vi "ChromaAcLoad.vi"() -> ()   [LabVIEW 2018, in "Visualization.lvlib" / "VisualizeAcPwr.lvclass"]
doc: "This VI listens for any measurement data associated with the provided PluginName and displays it to the user for analysis. The display is only suitable for data coming from the RoomAlert Plugin."
uses:
  VisualizeAcPwr.lvclass
  ChromaPowerSupply/Loop Parameters.ctl
  VisualizeBase/VisualizeBase_class/SubVIs/VisualizationOptions.ctl
  <vilib>/Utility/miscctls.llb/LVRectTypeDef.ctl
  AcPwr/AcPwrPlugins/ChromaAcLoadClass/TypeDefs/Device(s)Settings.ctl
  AcPwr/AcPwrPlugins/ChromaAcLoadClass/TypeDefs/ConfigMode.ctl
  AcPwr/AcPwrPlugins/ChromaAcLoadClass/TypeDefs/Measurements.ctl
  AcPwr/AcPwrPlugins/ChromaAcLoadClass/TypeDefs/MeasurementType.ctl
  AcPwr/AcPwrShared/clMeasurmentData.ctl
  AcPwr/AcPwrPlugins/AcPwrBaseClass/TypeDefs/SetParameterInputs.ctl
  <vilib>/event_ctls.llb/usereventprio.ctl
  VisualizeBase/VisualizeBase_class/Requests/VisUserEventType.ctl
  <extravilib>/ChannelInstances/Tag-bool/Write With Abort.vi
  <extravilib>/ChannelInstances/Tag-bool/Read With Abort.vi
  <extravilib>/ChannelInstances/Tag-bool/Instantiate.vi
  <extravilib>/ChannelInstances/Tag-bool/EndpointRead.vi
  <vilib>/Utility/error.llb/Error Cluster From Error Code.vi
  <extravilib>/ChannelInstances/Tag-bool/Endpoint.vi
  <vilib>/ErrorRing/Error Ring.xnode
  <userlib>/NIST/NISTErrorLib/NISTErrorLib.lvlib
  VisualizeBase/VisualizeBase_class/VisualizeBase.lvclass
  <extravilib>/ChannelInstances/Tag-bool.lvlib
  TestClass/Test.lvclass
  Sensor/VisualizeSensor.lvclass
  StatusAndLog/VisualizeStatus.lvclass
  AcPwr/AcPwrShared/AcPwrShared.lvlib
  AcPwr/AcPwrModule/AcPwrModule.lvlib
  AcPwr/AcPwrPlugins/ChromaAcLoadClass/ChromaAcLoad.lvclass
  AcPwr/AcPwrPlugins/AcPwrPlugins.lvlib
  AcPwr/AcPwrPlugins/AcPwrBaseClass/AcPwrBase.lvclass
panel:
  out "Chart#":i32
  out "MeasChannels":string[](array[string])
  out "Writetime":u32 caption="Sample Write Time(ms)"
  out "ExitHelperLoops?":bool
  out "CurrentType":string
  in  "Display":enum16{"Raw Data", "Voltage Vs Current"}(ring)
  in  "btnPause":bool
  in  "INIFilePath":path
  in  "ModuleID":i32
  in  "Log Data":bool=TRUE
  in  "btnStop":bool
  in  "btnReset":bool
  in  "btnClearTest":bool
  in  "btnStopModule":bool
  out "XY Graph":cluster{dbl[], dbl[]}(graph)
  out "Chart":waveform(dbl)[](graph)=[{"t0"=timestamp(3657200531.6397257 s since 1904-01-01), "dt"=1.0, "Y"=[46.19]}, {"t0"=timestamp(3657200531.6397257 s since 1904-01-01), "dt"=1.0, "Y"=[2.0]}, {"t0"=timestamp(3657200531.6397257 s since 1904-01-01), "dt"=1.0, "Y"=[60.0]}]
  in  "Device ON?":bool=TRUE
  in  "Resistance":bool
  in  "Power":bool
  in  "Current":bool
  in  "Voltage":bool
  in  "Resistance (Ohms)":dbl
  in  "Power (W)":dbl
  in  "Current (A)":dbl
  in  "Voltage (V)":dbl
  in  "btnRunParamLoop":bool
  in  "btnStopParameterLoop":bool
  in  "Loop Parameters":T1={"Parameter"=enum."Voltage", "Start Value"=5.0, "Increment"=1.0, "Interval (s)"=3.0, "# Iterations"=6, "End Value"=10.0} {"# Iterations" min=1; "Increment" format="%#.4f"}
  out "ErrorArray":errorcluster[](array[cluster])
  out "Incorrect DataType?":bool
  out "String Results":string
  in  "PluginName":string="Sensor.RoomAlert1"
  # "Set Parameter"
  # "Parameter Looping"
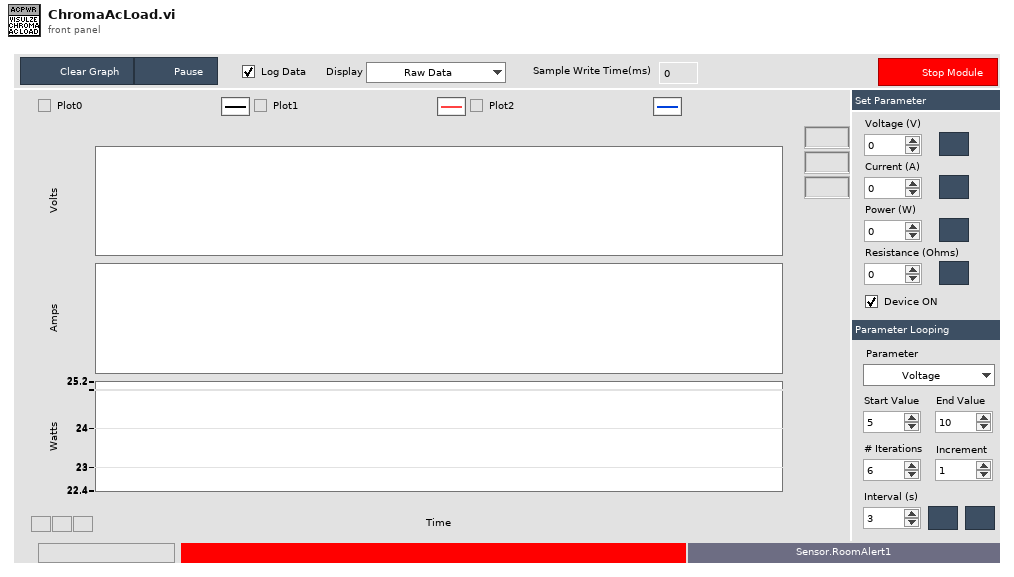
[diagram p1: front panel]
types:
  T1 = typedef "Loop Parameters.ctl" = cluster{"Parameter":enum16{"Voltage", "Current", "Power", "Resistance"}, "Start Value":dbl, "Increment":dbl, "Interval (s)":dbl, "# Iterations":u32, "End Value":dbl}
  T2 = typedef "Visualization.lvlib/VisualizeBase.lvclass/VisualizationOptions.ctl" = cluster{"PauseAtStartup":bool, "LogData":bool, "LaunchInSubPanel":bool, "FPMonitor":u16, "FPWindowBounds":T3, "MonitorBounds":cluster{"Left":i16, "Top":i16, "Right":i16, "Bottom":i16}, "MeasIndices":i32[]}
  T3 = typedef "LVRectTypeDef.ctl" = cluster{"Left":i16, "Top":i16, "Right":i16, "Bottom":i16}
  T4 = enum16{"open", "open or create", "create or replace", "create", "open (read-only)"}
  T5 = typedef "Visualization.lvlib/VisualizeBase.lvclass/VisRequestEvents.ctl" = cluster{"StopRequest":refnum<user-event>, "ResetRequest":refnum<user-event>, "FP Pop In or Out":refnum<user-event>}
  T6 = typedef "AcPwrShared.lvlib/AcPwrBroadcastEvents.ctl" = cluster{"DidInit":refnum<user-event>, "StatusUpdate":refnum<user-event>, "ErrorReport":refnum<user-event>, "DidStop":refnum<user-event>, "PathToINI":refnum<user-event>, "Measurements":refnum<user-event>, "LoadConfigFile":refnum<user-event>, "GetSettings":refnum<user-event>, "SetSettings":refnum<user-event>, "GetType&ID":refnum<user-event>, "GotSettings":refnum<user-event>, "GotSettingsLV":refnum<user-event>, "ParameterSet":refnum<user-event>}
  T7 = typedef "Visualization.lvlib/VisualizeBase.lvclass/VisFrmWrkBroadcastEvents.ctl" = cluster{"StatusUpdate":refnum<user-event>, "DidStop":refnum<user-event>, "NewModuleLoaded":refnum<user-event>, "StopVisualization":refnum<user-event>}
  T8 = typedef "AcPwrPlugins.lvlib/ChromaAcLoad.lvclass/Device(s)Settings.ctl" = cluster{"Configuration Mode":T9, "Phases":cluster{"Handle":string, "Name":string, "Phase Select":i32, "Instrument Options":string, "id query (T)":bool, "reset device (T)":bool, "Load Short Circuited":bool, "Line Synchronization":bool, "Load Current (A/Arms)":dbl, "Load Voltage (V/Vrms)":dbl, "Load Power (W)":dbl, "Load Resistance (Ohms)":dbl, "Load Current Peak Limit (A)":dbl, "Load Current Limit (A/Arms)":dbl, "Load Power Limit (W)":dbl, "Synch Frequency (Hz)":dbl, "Priority":enum16{"CF Only", "PF Only", "Both (CF)", "Both (PF)"}, "Crest Factor":dbl, "Power Factor":dbl, "Slew Rate":cluster{"Rise Slew Rate (A/ms)":i32, "Fall Slew Rate (A/ms)":i32}, "LC/RLC Mode":cluster{"Capacitance (uF)":i32, "Inductance (uH)":i32, "Series Resistance (Ohm)":dbl, "Parallel Resistance (Ohm)":dbl}, "Timing":cluster{"TimingOn":enum16{""}, "Hours":u32, "Minutes":u32, "Seconds":dbl, "CutoffVoltage":dbl}, "Connected":bool}[], "MeasName":string}
  T9 = typedef "AcPwrPlugins.lvlib/ChromaAcLoad.lvclass/ConfigMode.ctl" = enum16{"Constant Voltage (DC)", "Constant Power (DC)", "Constant Power (AC)", "Constant Current (DC)", "Constant Current (AC)", "Constant Resistance (DC)", "Constant Resistance (AC)", "Rectified Mode (DC)", "Inrush (AC)", "RLC CP (AC)", "RLC (AC)"}
  T10 = typedef "AcPwrPlugins.lvlib/ChromaAcLoad.lvclass/Measurements.ctl" = cluster{"Handle":string, "Name":string, "Enabled":bool, "Measurement Value":dbl, "Hold Peak Current Measurement":bool, "btnMeasFetch":bool, "ProtectionStatusString":string, "Measurement Type":T11}[]
  T11 = typedef "AcPwrPlugins.lvlib/ChromaAcLoad.lvclass/MeasurementType.ctl" = enum16{"Voltage (Vrms or V)", "Current (Arms or A)", "Power (W)", "Peak Voltage (V)", "Peak Current (A)", "Peak Power (W)", "Frequency (Hz)", "Resistance (Ohms)", "Voltage Overshoot (V)", "Positive Peak Current (A)", "Voltage Undershoot (V)", "Negative Peak Current (A)", "Apparent Power (VA)", "Reacitive Power (VAR)", "Voltage THD", "Power Factor", "Current's Crest Factor"}
  T12 = typedef "AcPwrShared.lvlib/clMeasurmentData.ctl" = cluster{"MeasName":string, "XML Data":string, "WaveformData":waveform(dbl)[]}
  T13 = typedef "AcPwrPlugins.lvlib/AcPwrBase.lvclass/SetParameterInputs.ctl" = cluster{"Type":string, "Parameter":string, "Phase":i32, "Value":dbl, "Command":string, "Time Stamp":timestamp}
  T14 = typedef "Visualization.lvlib/VisualizeBase.lvclass/VisUserEventType.ctl" = cluster{"BusIndex":i8, "Data":variant}
  T15 = typedef "usereventprio.ctl" = enum32{"high priority", "normal priority"}
  T16 = cluster{"Handle":string, "Name":string, "Phase Select":i32, "Instrument Options":string, "id query (T)":bool, "reset device (T)":bool, "Load Short Circuited":bool, "Line Synchronization":bool, "Load Current (A/Arms)":dbl, "Load Voltage (V/Vrms)":dbl, "Load Power (W)":dbl, "Load Resistance (Ohms)":dbl, "Load Current Peak Limit (A)":dbl, "Load Current Limit (A/Arms)":dbl, "Load Power Limit (W)":dbl, "Synch Frequency (Hz)":dbl, "Priority":enum16{"CF Only", "PF Only", "Both (CF)", "Both (PF)"}, "Crest Factor":dbl, "Power Factor":dbl, "Slew Rate":cluster{"Rise Slew Rate (A/ms)":i32, "Fall Slew Rate (A/ms)":i32}, "LC/RLC Mode":cluster{"Capacitance (uF)":i32, "Inductance (uH)":i32, "Series Resistance (Ohm)":dbl, "Parallel Resistance (Ohm)":dbl}, "Timing":cluster{"TimingOn":enum16{""}, "Hours":u32, "Minutes":u32, "Seconds":dbl, "CutoffVoltage":dbl}, "Connected":bool}[]
  T17 = cluster{"Handle":string, "Name":string, "Phase Select":i32, "Instrument Options":string, "id query (T)":bool, "reset device (T)":bool, "Load Short Circuited":bool, "Line Synchronization":bool, "Load Current (A/Arms)":dbl, "Load Voltage (V/Vrms)":dbl, "Load Power (W)":dbl, "Load Resistance (Ohms)":dbl, "Load Current Peak Limit (A)":dbl, "Load Current Limit (A/Arms)":dbl, "Load Power Limit (W)":dbl, "Synch Frequency (Hz)":dbl, "Priority":enum16{"CF Only", "PF Only", "Both (CF)", "Both (PF)"}, "Crest Factor":dbl, "Power Factor":dbl, "Slew Rate":cluster{"Rise Slew Rate (A/ms)":i32, "Fall Slew Rate (A/ms)":i32}, "LC/RLC Mode":cluster{"Capacitance (uF)":i32, "Inductance (uH)":i32, "Series Resistance (Ohm)":dbl, "Parallel Resistance (Ohm)":dbl}, "Timing":cluster{"TimingOn":enum16{""}, "Hours":u32, "Minutes":u32, "Seconds":dbl, "CutoffVoltage":dbl}, "Connected":bool}
  T18 = typedef "Tag-bool.lvlib/))Channel.ctl" = refnum<queue>
  T19 = typedef "sizeaction.ctl" = enum32{"Minimized", "Maximized", "Resized"}
  T20 = typedef "LVPoint32TypeDef.ctl" = cluster{"Horizontal":i32, "Vertical":i32}
  T21 = enum16{"Voltage", "Current", "Power", "Resistance"}
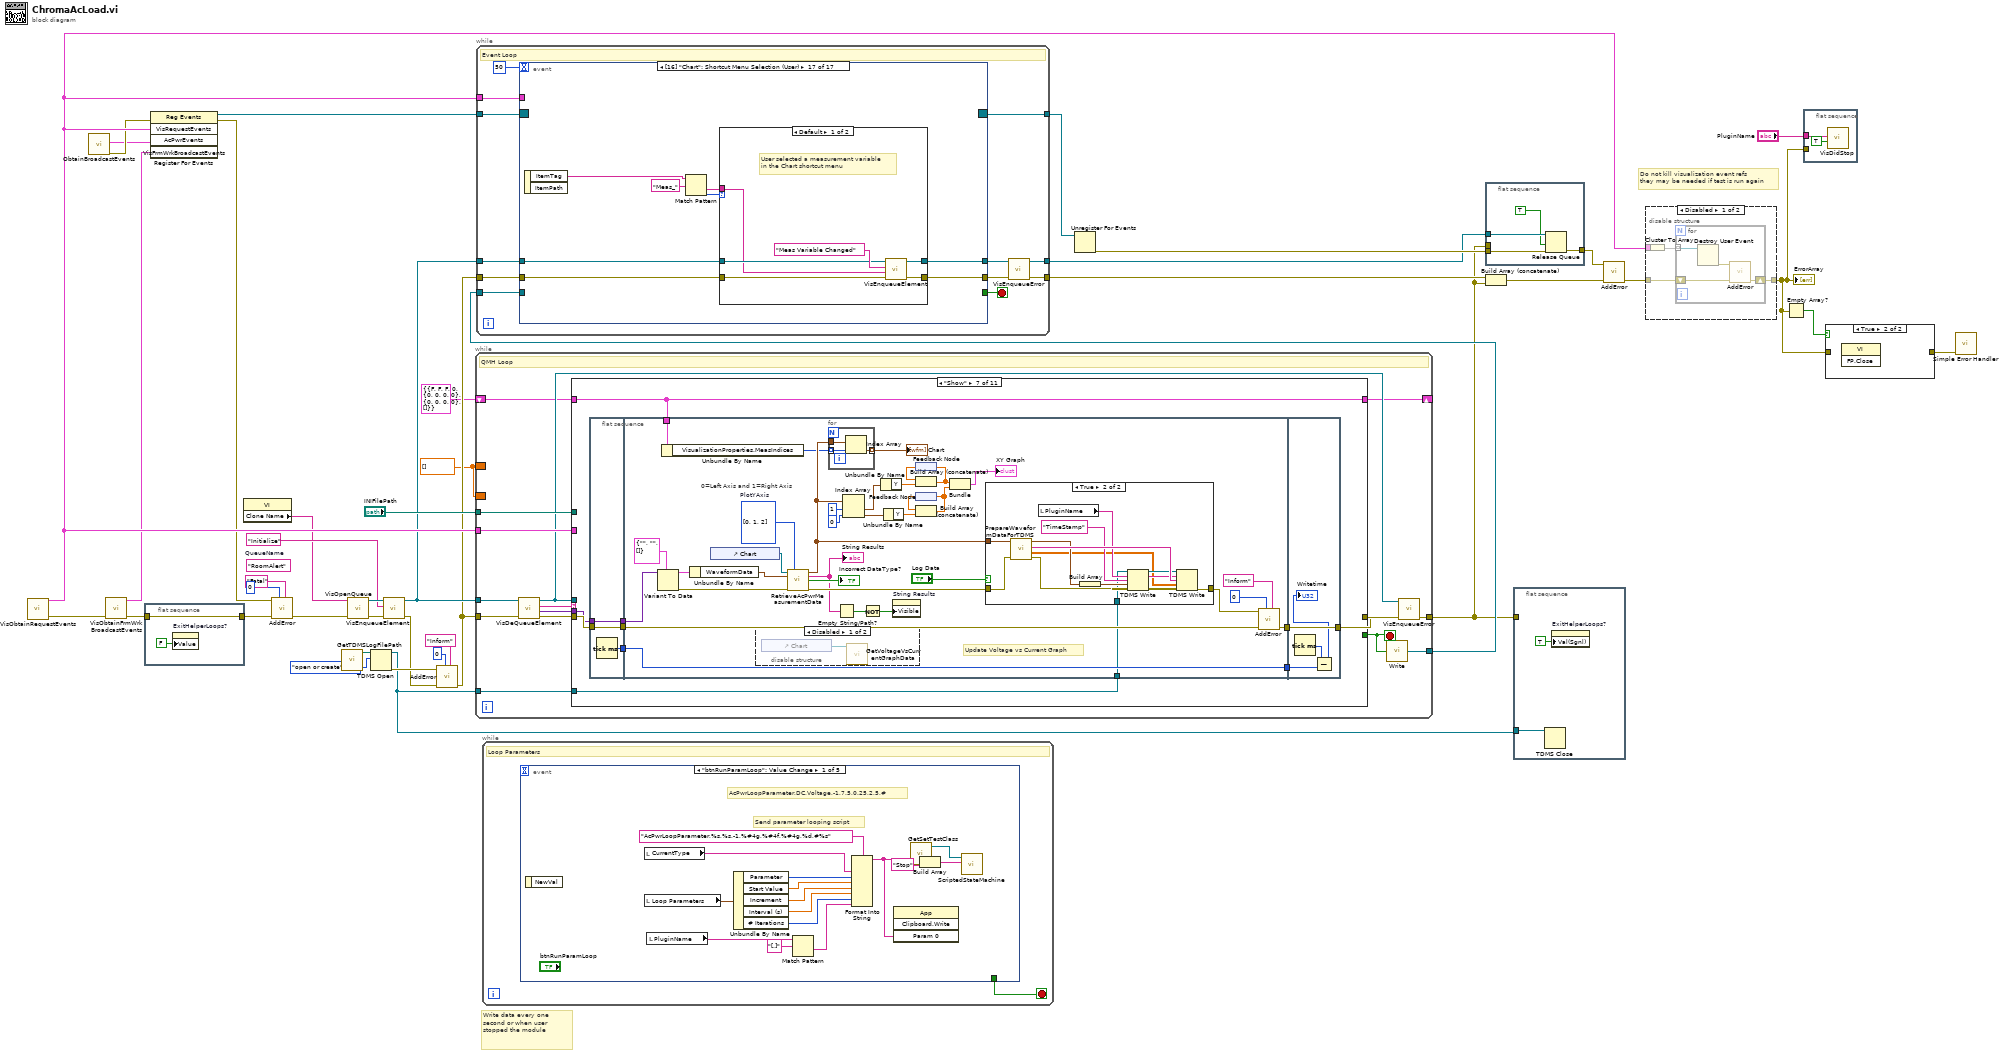
[diagram p0: block diagram]
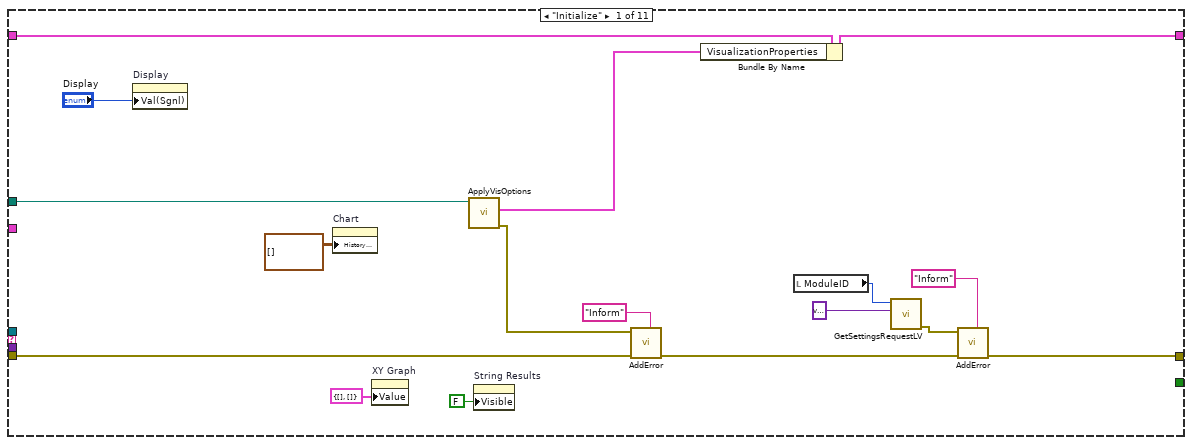
[diagram p2: hidden frame]
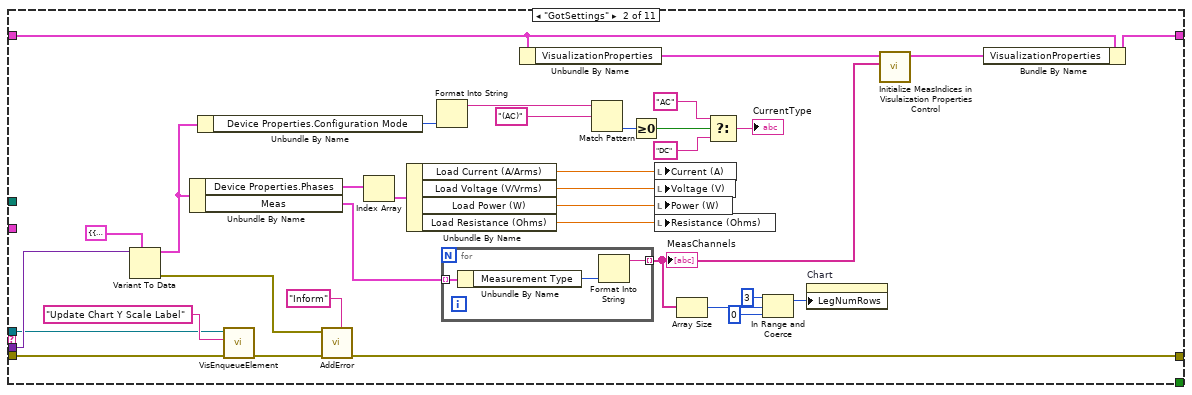
[diagram p3: hidden frame]
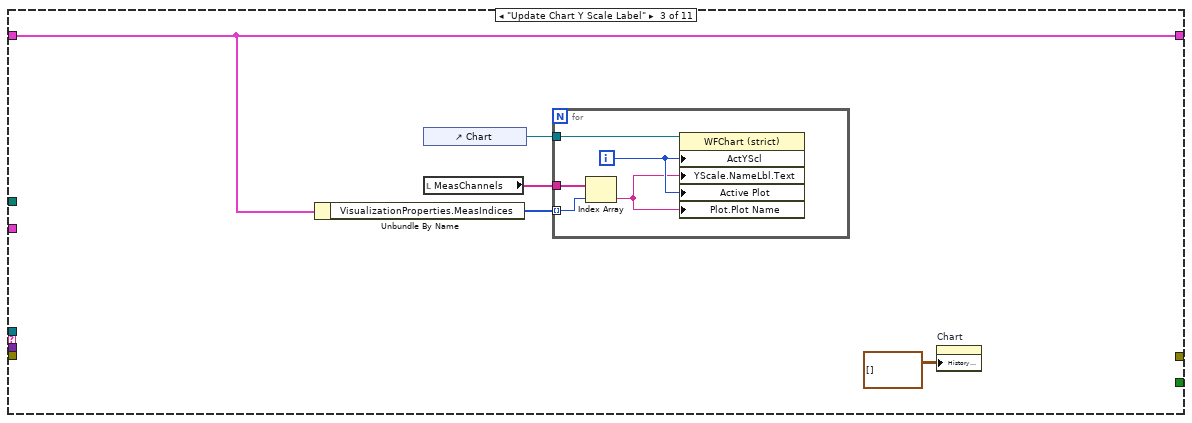
[diagram p4: hidden frame]
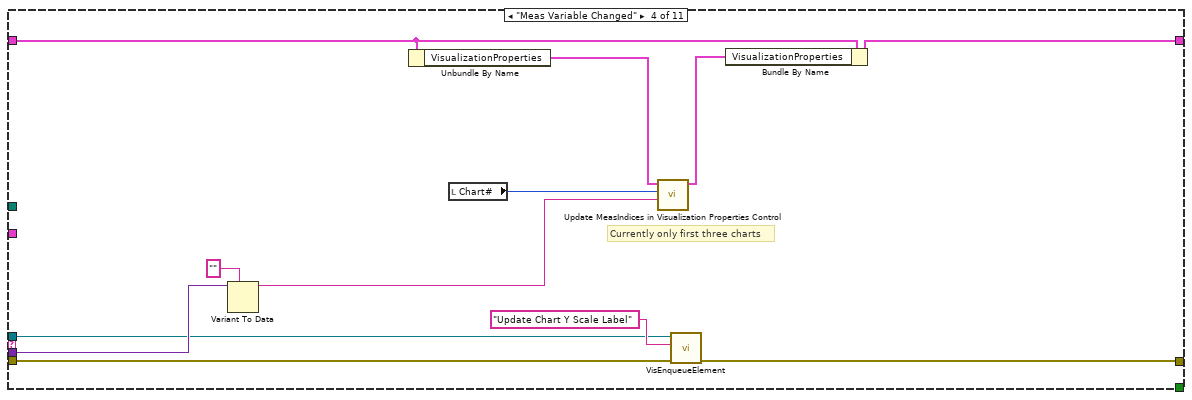
[diagram p5: hidden frame]
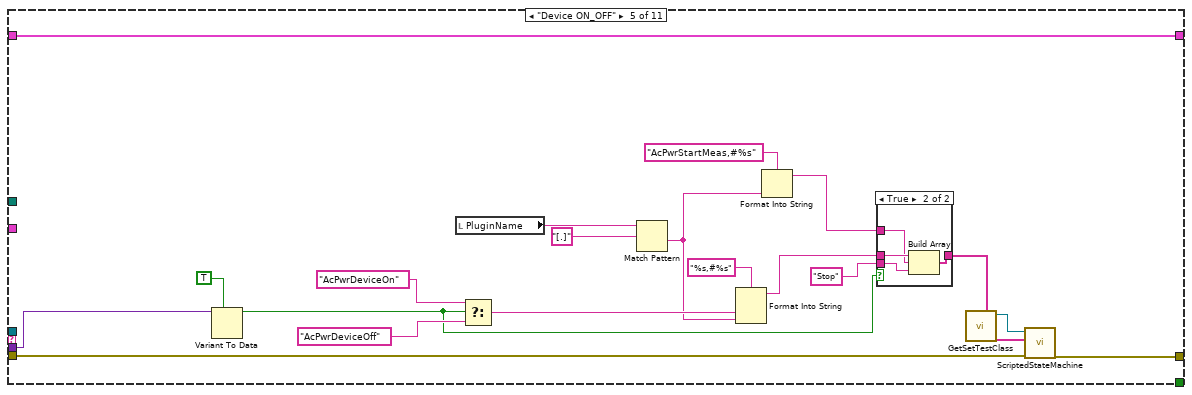
[diagram p6: hidden frame]
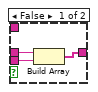
[diagram p7: hidden frame]
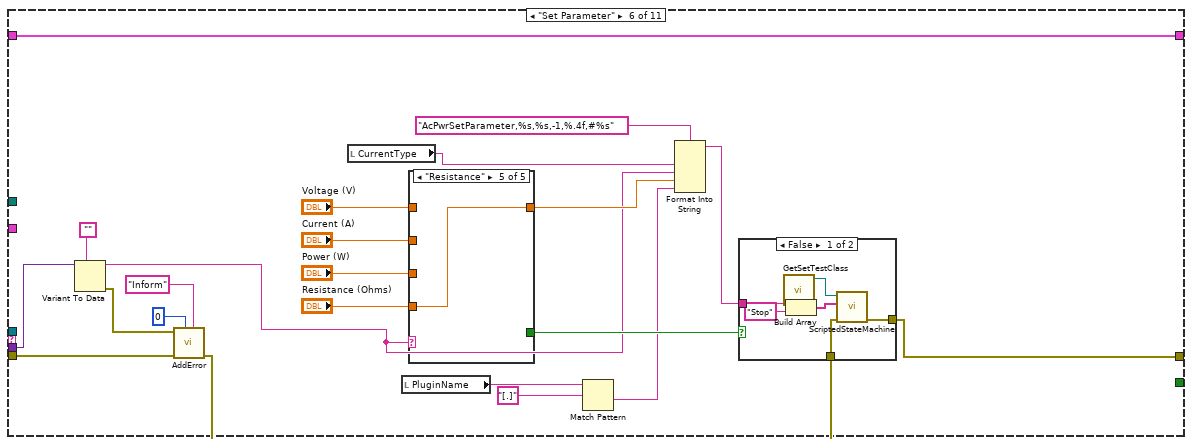
[diagram p8: hidden frame]
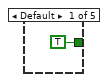
[diagram p10: hidden frame]
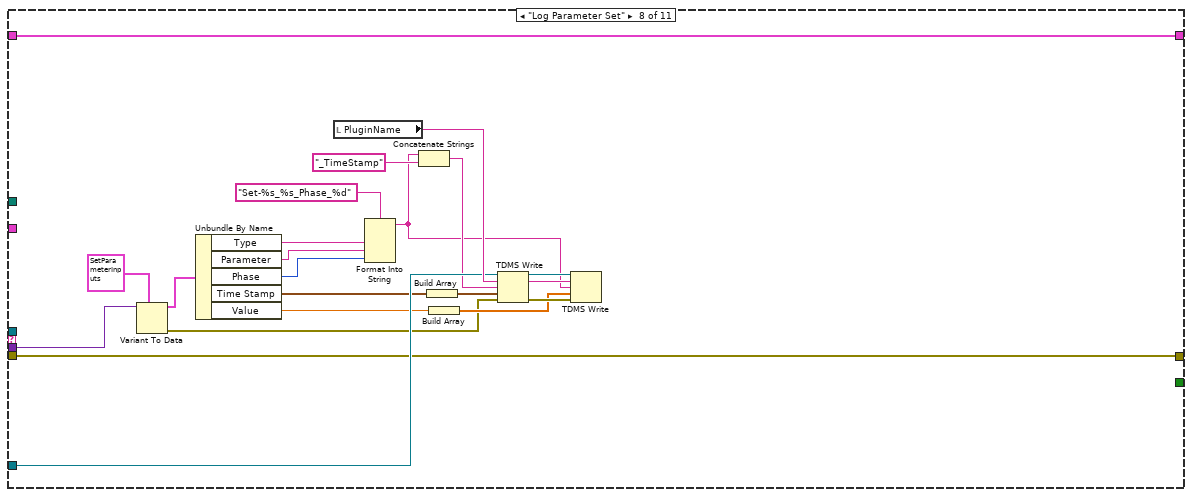
[diagram p16: hidden frame]
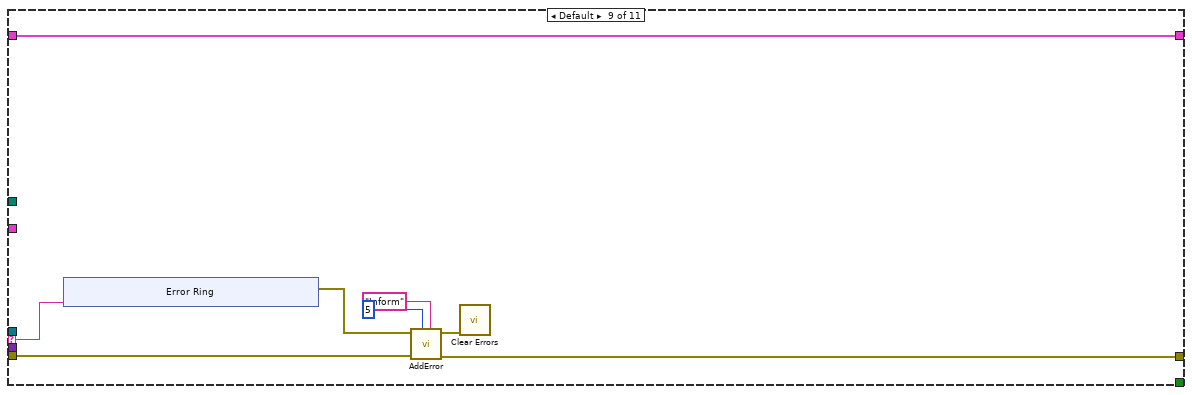
[diagram p17: hidden frame]
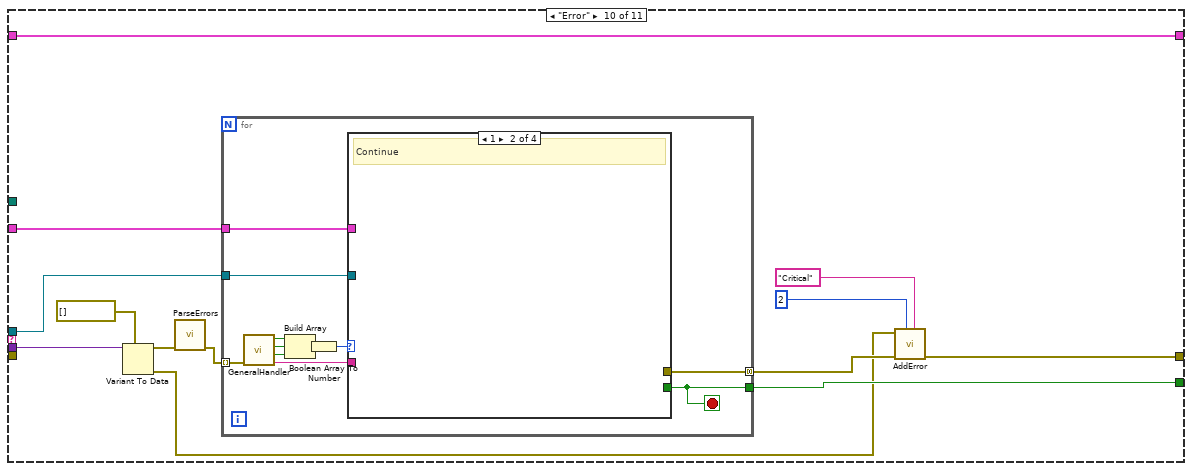
[diagram p18: hidden frame]
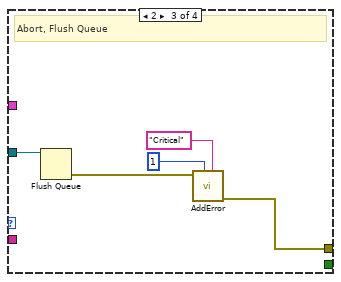
[diagram p20: hidden frame]
diagram:
  w3 = dbl[] []
  (unwired) "RoomAlert"  # QueueName
  # "Write data every one second or when user stopped the module"
  # "Do not kill visualization event refs\nthey may be needed if test is run again"
  n1 = call "VisObtainRequestEvents.vi"() -> ("Error"=w32:errorcluster[], "VisRequestEvents"=w34:T5)  [unwired: 10 in]
  n2 = call "ObtainBroadcastEvents.vi"() -> ("error out"=w28:errorcluster, "AcPwrEvents"=w21:T6)  [unwired: 10 in]
  n3 = call "VisObtainFrmWrkBroadcastEvents.vi"("Error"=w32) -> ("Error"=w7:errorcluster[], "VisFrmWrkBroadcastEvents"=w9:T7)  [unwired: 9 in]
  n4 = flat-sequence {
    tunnel: w7 -> [w42]
    tunnel: [w42] -> w6
    frame #0 {
      n5 = property on="ExitHelperLoops?" class="Bool (strict)"("Value"=FALSE ("ExitHelperLoops?")) -> ()  [unwired: 2 in, 2 out]
    }
  }
  n6 = register-events(error in=w28, w34, w21, w9) -> (reference out=w41:refnum<event-registration>, error out=w31:errorcluster)  [unwired: 1 in]
  n7 = property class="VI"() -> ("Clone Name"=w19:string)  [unwired: 2 in, 2 out]
  n8 = call <userlib>:"AddError.vi"("Severity"="Fatal", "Priority"=u8 0, "ErrorArray In"=w6, "error in (no error)"=w31) -> ("ErrorArray Out"=w27:errorcluster[])  [unwired: 6 in, 1 out]
  n9 = call "GetTDMSLogFilePath.vi"() -> ("TDMS Log File Path"=w18:path)  [unwired: 11 in]
  n10 = call "VisOpenQueue.vi"("Error Array In"=w27, "QueueName"=w19) -> ("Error Array Out"=w25:errorcluster[], "queue out"=w26:refnum<queue>)  [unwired: 8 in]
  n11 = TDMS Open(10:T4."open or create" ("operation (0:open)"), 11:w18) -> (0:w15:errorcluster, 3:w2:refnum<k34>)  [unwired: 5 in]
  n12 = call "VisEnqueueElement.vi"("Error Array In"=w25, "Message"="Initialize", "queue in"=w26) -> ("Error Array Out"=w5:errorcluster[], "queue out"=w8:refnum<queue>)  [unwired: 7 in]
  n13 = call <userlib>:"AddError.vi"("Severity"="Inform", "Priority"=u8 0, "ErrorArray In"=w5, "error in (no error)"=w15) -> ("ErrorArray Out"=w4:errorcluster[])  [unwired: 6 in, 1 out]
  n14 = while {
    tunnel: w4 -> [w52]
    tunnel: [w55] -> w13
    tunnel: w8 -> [w51]
    tunnel: w34 -> [w57]
    tunnel: [w49] -> w20
    tunnel: "INIFilePath" -> [w48]
    tunnel: w2 -> [w47]
    border: w3 -> [_]
    border: w3 -> [_]
    shift-right: [w44] -> _
    shift-left: cluster{"VisualizationProperties":T2} {"VisualizationProperties"={"PauseAtStartup"=FALSE, "LogData"=FALSE, "LaunchInSubPanel"=FALSE, "FPMonitor"=0, "FPWindowBounds"={"Left"=0, "Top"=0, "Right"=0, "Bottom"=0}, "MonitorBounds"={"Left"=0, "Top"=0, "Right"=0, "Bottom"=0}, "MeasIndices"=[]}} ("output cluster") -> [w45]
    stop <- w58 stop-if-true
    # "QMH Loop"
    n15 = call "VisDeQueueElement.vi"("Error Array In"=w52, "Queue In"=w51) -> ("Error Array Out"=w50:errorcluster[], "Data"=w53:variant, "Message"=w54:string, "Queue Out"=w46:refnum<queue>)  [unwired: 6 in]
    n16 = case shown="\"Show\"" w54 {
      selector: w54 -> [_ _ _ _ _ _ _ _ w295 _ _]
      tunnel: w53 -> [_ w109 _ w128 w143 w165 w202 w287 _ w315 _]
      tunnel: w50 -> [w72 w86 _ w124 w141 w166 w203 w267 w293 _ w345]
      tunnel: [w65 w85 _ w123 w140 w162 w204 w267 w292 w306 w344] -> w56
      tunnel: [_ _ _ _ _ _ _ _ _ w311 TRUE] -> w58
      tunnel: w57 -> [_ _ _ _ _ _ _ _ _ w310 _]
      tunnel: w48 -> [w71 _ _ _ _ _ _ _ _ _ w346]
      tunnel: w47 -> [_ _ _ _ _ _ w196 w276 _ _ _]
      tunnel: w46 -> [_ w88 _ w125 _ _ _ _ _ w304 _]
      tunnel: w45 -> [w61 w84 w113 w133 w135 w161 w195 w266 w288 w303 w343]
      tunnel: [w60 w82 w113 w131 w135 w161 w195 w266 w288 w303 w343] -> w44
      frame "Initialize" {
        n17 = property on="Display" class="Enum (strict)"("Val(Sgnl)"="Display") -> ()  [unwired: 2 in, 2 out]
        n18 = property on="Chart" class="WFChart (strict)"("History Data"=waveform(dbl)[][] []) -> ()  [unwired: 2 in, 2 out]
        n19 = property on="XY Graph" class="XYGraph (strict)"("Value"=cluster{dbl[], dbl[]} {[], []} ("XY Graph")) -> ()  [unwired: 2 in, 2 out]
        n20 = call "ApplyVisOptions.vi"("INIFilePath"=w71) -> ("error out"=w75:errorcluster, "VisualizationProperties"=w59:T2)  [unwired: 9 in]
        n21 = property on="String Results" class="Str"("Visible"=FALSE) -> ()  [unwired: 2 in, 2 out]
        n22 = call <userlib>:"AddError.vi"("Severity"="Inform", "ErrorArray In"=w72, "error in (no error)"=w75) -> ("ErrorArray Out"=w73:errorcluster[])  [unwired: 7 in, 1 out]
        n23 = Bundle By Name(cluster=w61, "VisualizationProperties"=w59) -> (w60:cluster{"VisualizationProperties":T2})
        n24 = local read "ModuleID"() -> (w67:i32)
        n25 = call "GetSettingsRequestLV.vi"("SettingsToGet"=variant, "ModuleID"=w67) -> ("Error Out"=w64:errorcluster)  [unwired: 9 in]
        n26 = call <userlib>:"AddError.vi"("Severity"="Inform", "ErrorArray In"=w73, "error in (no error)"=w64) -> ("ErrorArray Out"=w65:errorcluster[])  [unwired: 7 in, 1 out]
      }
      frame "GotSettings" {
        n27 = Variant To Data(type=cluster{"Device Properties":T8, "Meas":T10} {"Device Properties"={"Configuration Mode"=enum."Constant Voltage (DC)", "Phases"=[], "MeasName"=""}, "Meas"=[]} ("output cluster"), Variant=w109) -> (data=w99:cluster{"Device Properties":T8, "Meas":T10}, error out=w101:errorcluster)  [unwired: 1 in]
        n28 = Unbundle By Name(w99) -> ("Device Properties.Phases"=w107:T16, "Meas"=w90:T10)
        n29 = Unbundle By Name(w99) -> ("Device Properties.Configuration Mode"=w98:T9)
        n30 = call "VisEnqueueElement.vi"("Error Array In"=w86, "Message"="Update Chart Y Scale Label", "queue in"=w88) -> ("Error Array Out"=w87:errorcluster[])  [unwired: 7 in, 1 out]
        n31 = call <userlib>:"AddError.vi"("Severity"="Inform", "ErrorArray In"=w87, "error in (no error)"=w101) -> ("ErrorArray Out"=w85:errorcluster[])  [unwired: 7 in, 1 out]
        n32 = Index Array(array=w107) -> (element=w106:T17)  [unwired: 1 in]
        n33 = Unbundle By Name(w106) -> ("Load Current (A/Arms)"=w105:dbl, "Load Voltage (V/Vrms)"=w104:dbl, "Load Power (W)"=w103:dbl, "Load Resistance (Ohms)"=w102:dbl)
        n34 = Format Into String(w98) -> (resulting string=w97:string)  [unwired: 3 in, 1 out]
        n35 = for {
          tunnel: w90 -> [w112] mode=indexing
          tunnel: [w110] -> w80 mode=indexing
          n36 = Unbundle By Name(w112) -> ("Measurement Type"=w111:T11)
          n37 = Format Into String(w111) -> (resulting string=w110:string)  [unwired: 3 in, 1 out]
        }
        "MeasChannels" <- w80
        n38 = Unbundle By Name(w84) -> ("VisualizationProperties"=w83:T2)
        n39 = Match Pattern(string=w97, regular expression="(AC)") -> (offset past match=w95:i32)  [unwired: 1 in, 3 out]
        n40 = Greater Or Equal To 0?(x=w95) -> (x >= 0?=w94:bool)
        n41 = local write "Current (A)"(w105) -> ()
        n42 = local write "Voltage (V)"(w104) -> ()
        n43 = local write "Power (W)"(w103) -> ()
        n44 = local write "Resistance (Ohms)"(w102) -> ()
        n45 = Array Size(array=w80) -> (size(s)=w79:i32)
        n46 = Select(t="AC" ("regular expression"), s=w94, f="DC" ("regular expression")) -> (s? t:f=→"CurrentType":string)
        n47 = In Range and Coerce(upper limit=3, x=w79, lower limit=0) -> (coerced(x)=w76:i32)  [unwired: 1 out]
        n48 = property on="Chart" class="WFChart (strict)"("LegNumRows"=w76) -> ()  [unwired: 2 in, 2 out]
        n49 = call "Initialize MeasIndices in Visulaization Properties Control.vi"("MeasChannels"=w80, "VisualizationProperties"=w83) -> ("VisualizationProperties out"=w81:T2)  [unwired: 8 in, 1 out]
        n50 = Bundle By Name(cluster=w84, "VisualizationProperties"=w81) -> (w82:cluster{"VisualizationProperties":T2})
      }
      frame "Update Chart Y Scale Label" {
        n51 = Unbundle By Name(w113) -> ("VisualizationProperties.MeasIndices"=w114:i32[])
        n52 = control-ref of="Chart"() -> (w116:refnum<vi>)
        n53 = local read "MeasChannels"() -> (w115:string[])
        n54 = for {
          tunnel: w114 -> [w120] mode=indexing
          tunnel: w116 -> [w122]
          tunnel: w115 -> [w121]
          i -> [w119]
          n55 = Index Array(array=w121, index=w120) -> (element=w118:string)
          n56 = property class="WFChart (strict)"(reference=w122, "ActYScl"=w119, "YScale.NameLbl.Text"=w118, "Active Plot"=w119, "Plot.Plot Name"=w118) -> ()  [unwired: 1 in, 2 out]
        }
        n57 = property on="Chart" class="WFChart (strict)"("History Data"=waveform(dbl)[][] []) -> ()  [unwired: 2 in, 2 out]
      }
      frame "Meas Variable Changed" {
        # "Currently only first three charts"
        n58 = Variant To Data(type="" ("Message"), Variant=w128) -> (data=w127:string)  [unwired: 1 in, 1 out]
        n59 = Unbundle By Name(w133) -> ("VisualizationProperties"=w132:T2)
        n60 = local read "Chart#"() -> (w134:i32)
        n61 = call "Update MeasIndices in Visualization Properties Control.vi"("Item Tag"=w127, "Chart# user clicked on"=w134, "VisualizationProperties In"=w132) -> ("VisualizationProperties"=w130:T2)  [unwired: 8 in]
        n62 = call "VisEnqueueElement.vi"("Error Array In"=w124, "Message"="Update Chart Y Scale Label", "queue in"=w125) -> ("Error Array Out"=w123:errorcluster[])  [unwired: 7 in, 1 out]
        n63 = Bundle By Name(cluster=w133, "VisualizationProperties"=w130) -> (w131:cluster{"VisualizationProperties":T2})
      }
      frame "Device ON_OFF" {
        n64 = Variant To Data(type=TRUE, Variant=w143) -> (data=w137:bool)  [unwired: 1 in, 1 out]
        n65 = local read "PluginName"() -> (w149:string)
        n66 = Select(t="AcPwrDeviceOn" ("format string"), s=w137, f="AcPwrDeviceOff" ("format string")) -> (s? t:f=w153:string)
        n67 = Match Pattern(string=w149, regular expression="[.]") -> (after substring=w138:string)  [unwired: 1 in, 3 out]
        n68 = Format Into String(format string="%s,#%s", w153, w138) -> (resulting string=w150:string)  [unwired: 2 in, 1 out]
        n69 = Format Into String(format string="AcPwrStartMeas,#%s", w138) -> (resulting string=w136:string)  [unwired: 2 in, 1 out]
        n70 = case shown="True" w137 {
          tunnel: [w156 w157] -> w152
          tunnel: w150 -> [w155 w160]
          tunnel: "Stop" ("element") -> [w154 w158]
          tunnel: w136 -> [_ w159]
          frame False {
            n71 = Build Array(w155, w154) -> (w156:string[])
          }
          frame True {
            n72 = Build Array(w160, w159, w158) -> (w157:string[])
          }
        }
        n73 = call "GetSetTestClass.vi"() -> ("Test.lvclass"=w151:refnum<class "Test.lvclass">)  [unwired: 11 in]
        n74 = call "ScriptedStateMachine.vi"("ErrorArray 2"=w141, "script"=w152, "Test.lvclass 2"=w151) -> ("ErrorArray"=w140:errorcluster[])  [unwired: 6 in, 2 out]
      }
      frame "Set Parameter" {
        n75 = Variant To Data(type="", Variant=w165) -> (data=w164:string, error out=w168:errorcluster)  [unwired: 1 in]
        n76 = call <userlib>:"AddError.vi"("Severity"="Inform", "Priority"=u8 0, "ErrorArray In"=w166, "error in (no error)"=w168) -> ("ErrorArray Out"=w163:errorcluster[])  [unwired: 6 in, 1 out]
        n77 = local read "CurrentType"() -> (w182:string)
        n78 = local read "PluginName"() -> (w178:string)
        n79 = case shown="\"Resistance\"" w164 {
          tunnel: "Voltage (V)" -> [_ w191 _ _ _]
          tunnel: "Current (A)" -> [_ _ w192 _ _]
          tunnel: "Power (W)" -> [_ _ _ w193 _]
          tunnel: "Resistance (Ohms)" -> [_ _ _ _ w194]
          tunnel: [_ w191 w192 w193 w194] -> w177
          tunnel: [TRUE _ _ _ _] -> w180
          frame Default {
          }
          frame "Voltage" {
          }
          frame "Current" {
          }
          frame "Power" {
          }
          frame "Resistance" {
          }
        }
        n80 = Match Pattern(string=w178, regular expression="[.]") -> (after substring=w179:string)  [unwired: 1 in, 3 out]
        n81 = Format Into String(format string="AcPwrSetParameter,%s,%s,-1,%.4f,#%s", w182, w164, w177, w179) -> (resulting string=w181:string)  [unwired: 2 in, 1 out]
        n82 = case shown="False" w180 {
          tunnel: w181 -> [w187 _]
          tunnel: [w185 w189] -> w162
          tunnel: w163 -> [w183 w189]
          frame False {
            n83 = call "GetSetTestClass.vi"() -> ("Test.lvclass"=w188:refnum<class "Test.lvclass">)  [unwired: 11 in]
            n84 = Build Array(w187, "Stop" ("element")) -> (w186:string[])
            n85 = call "ScriptedStateMachine.vi"("ErrorArray 2"=w183, "script"=w186, "Test.lvclass 2"=w188) -> ("ErrorArray"=w185:errorcluster[])  [unwired: 6 in, 2 out]
          }
          frame True {
          }
        }
      }
      frame "Show" {
        n86 = flat-sequence {
          tunnel: w202 -> [w206]
          tunnel: w203 -> [w207]
          tunnel: [w207] -> w201
          tunnel: [w206] -> w200
          tunnel: [w205] -> w198
          tunnel: w201 -> [w241]
          tunnel: w200 -> [w238]
          tunnel: [w242] -> w199
          tunnel: w198 -> [w230]
          tunnel: [w230] -> w197
          tunnel: w196 -> [w226]
          tunnel: w195 -> [w208]
          tunnel: [w265] -> w204
          tunnel: w199 -> [w265]
          tunnel: w197 -> [w263]
          frame #0 {
            n87 = Tick Count (ms)() -> (millisecond timer value=w205:u32)
          }
          frame #1 {
            w235 = u32[] [0, 1, 2]  # PlotYAxis
            # "Update Voltage vs Current Graph"
            # "0=Left Axis and 1=Right Axis"
            n88 = Variant To Data(type=T12 {"MeasName"="", "XML Data"="", "WaveformData"=[]} ("MeasurmentDataCluster"), Variant=w238) -> (data=w236:T12, error out=w237:errorcluster)  [unwired: 1 in]
            n89 = Unbundle By Name(w208) -> ("VisualizationProperties.MeasIndices"=w209:i32[])
            n90 = Unbundle By Name(w236) -> ("WaveformData"=w232:waveform(dbl)[])
            n91 = control-ref of="Chart"() -> (w231:refnum<vi>)
            n92 = disable-structure shown="Disabled" {
              frame Disabled {
                n93 = control-ref of="Chart"() -> (w246:refnum<vi>)
                n94 = call "GetVoltageVsCurrentGraphData.vi"("WaveformChart in"=w246) -> ()  [unwired: 9 in, 2 out]
              }
              frame Enabled {
              }
            }
            n95 = call "RetrieveAcPwrMeasurementData.vi"("WaveformChartReference"=w231, "PlotYScale"=w235, "WaveformArrayIn"=w232, "error in (no error)"=w237) -> ("WaveformArrayOut"=w211:waveform(dbl)[], "OutputString(Chroma)"=w214:string, "Incorrect DataType?"=→"Incorrect DataType?":bool, "error out"=w229:errorcluster)  [unwired: 7 in, 1 out]
            "String Results" <- w214
            n96 = for {
              tunnel: w211 -> [w245]
              tunnel: w209 -> [w244] mode=indexing
              tunnel: [w243] -> w210 mode=indexing
              n97 = Index Array(array=w245, index=w244) -> (element=w243:waveform(dbl))
            }
            "Chart" <- w210
            n98 = Empty String/Path?(string/path=w214) -> (empty?=w213:bool)
            n99 = Index Array(array=w211, index #1=1 ("index"), index #2=0 ("index")) -> (element #1=w216:waveform(dbl), element #2=w217:waveform(dbl))
            n100 = Not(x=w213) -> (.not. x?=w212:bool)
            n101 = Unbundle By Name(w216) -> ("Y"=w218:dbl[])
            n102 = Unbundle By Name(w217) -> ("Y"=w221:dbl[])
            n103 = property on="String Results" class="Str"("Visible"=w212) -> ()  [unwired: 2 in, 2 out]
            n104 = feedback #1() -> (w219:dbl[])
            n105 = Build Array (concatenate)(w219, w218) -> (w224:dbl[])
            n106 = feedback-in #1(w224) -> ()
            n107 = feedback #2() -> (w220:dbl[])
            n108 = Build Array (concatenate)(w220, w221) -> (w225:dbl[])
            n109 = feedback-in #2(w225) -> ()
            n110 = Bundle(w224, w225) -> (→"XY Graph":cluster{dbl[], dbl[]})  [unwired: 1 in]
            n111 = case shown="True" "Log Data" {
              tunnel: [w247 w261] -> w228
              tunnel: w229 -> [w247 w260]
              tunnel: w211 -> [_ w249]
              tunnel: w226 -> [_ w248]
              frame False {
              }
              frame True {
                n112 = call "PrepareWaveformDataForTDMS.vi"("error in (no error)"=w260, "WaveformArray in"=w249) -> ("error out"=w259:errorcluster, "Measurement Data"=w251:dbl[][], "Channel Names"=w258:string[], "TimeStamp"=w252:timestamp)  [unwired: 6 in]
                n113 = local read "PluginName"() -> (w255:string)
                n114 = Build Array(w252) -> (w250:timestamp[])
                n115 = TDMS Write(0:w248, 5:w255, 7:"TimeStamp" ("PluginName"), 9:w250, 11:w259) -> (4:w256:refnum<k34>, 6:w254:string, 15:w257:errorcluster)  [unwired: 1 in, 1 out]
                n116 = TDMS Write(0:w256, 5:w254, 7:w258, 9:w251, 11:w257) -> (15:w261:errorcluster)  [unwired: 1 in, 3 out]
              }
            }
            n117 = call <userlib>:"AddError.vi"("Severity"="Inform" ("String"), "Priority"=u8 0, "ErrorArray In"=w241, "error in (no error)"=w228) -> ("ErrorArray Out"=w242:errorcluster[])  [unwired: 6 in, 1 out]
          }
          frame #2 {
            n118 = Tick Count (ms)() -> (millisecond timer value=w264:u32)
            n119 = Subtract(x=w264, y=w263) -> (x-y=→"Writetime":u32)
          }
        }
      }
      frame "Log Parameter Set" {
        n120 = Variant To Data(type=T13 {"Type"="", "Parameter"="", "Phase"=0, "Value"=0.0, "Command"="", "Time Stamp"=timestamp(0 s since 1904-01-01)}, Variant=w287) -> (data=w280:T13, error out=w268:errorcluster)  [unwired: 1 in]
        n121 = Unbundle By Name(w280) -> ("Type"=w279:string, "Parameter"=w278:string, "Phase"=w277:i32, "Time Stamp"=w272:timestamp, "Value"=w270:dbl)
        n122 = local read "PluginName"() -> (w283:string)
        n123 = Format Into String(format string="Set-%s_%s_Phase_%d", w279, w278, w277) -> (resulting string=w271:string)  [unwired: 2 in, 1 out]
        n124 = Concatenate Strings(w271, "_TimeStamp" ("string")) -> (w273:string)
        n125 = Build Array(w272) -> (w281:timestamp[])
        n126 = Build Array(w270) -> (w269:dbl[])
        n127 = TDMS Write(0:w276, 5:w283, 7:w273, 9:w281, 11:w268) -> (4:w284:refnum<k34>, 6:w282:string, 15:w285:errorcluster)  [unwired: 1 in, 1 out]
        n128 = TDMS Write(0:w284, 5:w282, 7:w271, 9:w269, 11:w285) -> ()  [unwired: 1 in, 4 out]
      }
      frame Default {
        n129 = xnode "Error Ring"("parameter 0"=w295) -> ("error out"=w294:errorcluster)
        n130 = call <userlib>:"AddError.vi"("Severity"="Inform" ("String"), "Priority"=u8 5, "ErrorArray In"=w293, "error in (no error)"=w294) -> ("ErrorArray Out"=w292:errorcluster[], "error out"=w291:errorcluster)  [unwired: 6 in]
        n131 = call <vilib>:"Clear Errors.vi"("error in (no error)"=w291) -> ()  [unwired: 5 in, 2 out]
      }
      frame "Error" {
        n132 = Variant To Data(type=errorcluster[] [], Variant=w315) -> (data=w313:errorcluster[], error out=w305:errorcluster)  [unwired: 1 in]
        n133 = call <userlib>:"ParseErrors.vi"("ErrorArray"=w313) -> ("ErrorArray"=w312:errorcluster[])  [unwired: 8 in, 2 out]
        n134 = for {
          tunnel: w312 -> [w326] mode=indexing
          tunnel: [w320] -> w307 mode=concatenating
          tunnel: [w318] -> w311
          tunnel: w310 -> [w317]
          tunnel: w304 -> [w316]
          stop <- w318 stop-if-true
          n135 = call <userlib>:"GeneralHandler.vi"("error in (no error)"=w326) -> ("Severity"=w319:string, "Stop"=w323:bool, "Abort"=w324:bool, "Continue"=w325:bool)  [unwired: 6 in, 1 out]
          n136 = Build Array(w325, w324, w323) -> (w322:bool[])
          n137 = Boolean Array To Number(Boolean array=w322) -> (number=w321:u32)
          n138 = case shown="1" w321 {
            tunnel: [_ _ w331 w340] -> w320
            tunnel: w319 -> [_ _ _ w333]
            tunnel: [_ _ _ w335] -> w318
            tunnel: w317 -> [_ _ _ w334]
            tunnel: w316 -> [_ _ w327 _]
            frame 0, Default {
              # "No Dialog"
            }
            frame 1 {
              # "Continue"
            }
            frame 2 {
              # "Abort, Flush Queue"
              n139 = Flush Queue(queue=w327) -> (error out=w330:errorcluster)  [unwired: 1 in, 2 out]
              n140 = call <userlib>:"AddError.vi"("Severity"="Critical" ("String"), "Priority"=u8 1, "error in (no error)"=w330) -> ("ErrorArray Out"=w331:errorcluster[])  [unwired: 7 in, 1 out]
            }
            frame 4 {
              # "Stop"
              n141 = Unbundle By Name(w334) -> ("StopRequest"=w341:refnum<user-event>)
              n142 = Equal?(x=w333, y="Fatal" ("x")) -> (x = y?=w335:bool)
              n143 = Generate User Event(priority (normal)=usereventprio."high priority", user event=w341, event data cluster=T14 {"BusIndex"=0, "Data"=variant} ("event data")) -> (error out=w339:errorcluster)  [unwired: 1 in, 1 out]
              n144 = call <userlib>:"AddError.vi"("error in (no error)"=w339) -> ("ErrorArray Out"=w340:errorcluster[], "error out"=w336:errorcluster)  [unwired: 9 in]
              n145 = call <vilib>:"Clear Errors.vi"("error in (no error)"=w336) -> ()  [unwired: 5 in, 2 out]
            }
          }
        }
        n146 = call <userlib>:"AddError.vi"("Severity"="Critical", "Priority"=u8 2, "ErrorArray In"=w307, "error in (no error)"=w305) -> ("ErrorArray Out"=w306:errorcluster[])  [unwired: 6 in, 1 out]
      }
      frame "Stop" {
        n147 = Unbundle By Name(w343) -> ("VisualizationProperties"=w342:T2)
        n148 = call "WriteVisOptionsToINIFile.vi"("Visualization Options"=w342, "INIFilePath"=w346) -> ("error out"=w347:errorcluster)  [unwired: 8 in, 1 out]
        n149 = call <userlib>:"AddError.vi"("Severity"="Inform", "ErrorArray In"=w345, "error in (no error)"=w347) -> ("ErrorArray Out"=w344:errorcluster[])  [unwired: 7 in, 1 out]
      }
    }
    n150 = call <extravilib>:"Write.vi"("element"=w58) -> ("channel"=w49:T18)  [unwired: 1 out]
    n151 = call "VisEnqueueError.vi"("Error Array In"=w56, "Queue in"=w46) -> ("Error Array Out"=w55:errorcluster[])  [unwired: 8 in, 1 out]
  }
  n152 = while {
    tunnel: w41 -> [w361]
    tunnel: [w355] -> w39
    tunnel: [w359] -> w40
    tunnel: w34 -> [w358]
    tunnel: w4 -> [w357]
    tunnel: w8 -> [w356]
    tunnel: [w352] -> w23
    tunnel: w20 -> [w350]
    stop <- w360 stop-if-true
    # "Event Loop"
    n153 = event shown="[16] \"Chart\": Shortcut Menu Selection (User)" {
      selector: w361 -> [w364 w382 _ _ _ _ w438 w467 _ _ _ _ _ _ _ _ _]
      dyn-events: [w364 w381 _ _ _ _ w438 w467 _ _ _ _ _ _ _ _ _] -> w359
      timeout: 50 -> [_ _ _ _ _ _ _ _ _ _ _ _ _ _ _ _ _]
      tunnel: [_ _ FALSE ("Priority? (F)") _ _ w407 w435 w464 _ _ _ _ _ _ _ _ _] -> w360
      tunnel: [w367 w379 w386 w395 w402 w409 w440 w469 w502 _ w520 _ w532 w550 w557 w575 w585] -> w354
      tunnel: w358 -> [_ _ w385 _ _ _ _ _ _ _ _ _ _ _ _ _ _]
      tunnel: w357 -> [w368 w380 w393 _ _ w412 w441 w470 w501 _ _ _ w534 _ w558 w575 w583]
      tunnel: w356 -> [w363 w372 w383 w394 w401 w411 w442 w471 w504 w514 w521 w528 w535 w546 w559 w576 w584]
      tunnel: [w363 w372 w383 w394 w401 w410 w439 w468 w503 w514 w522 w527 w533 w546 w556 w576 w586] -> w353
      tunnel: w350 -> [_ _ _ _ _ w414 w436 w465 _ _ _ _ _ _ _ _ _]
      event "btnClearTest": Value Change {
        # "Erases the measurements on the graph."
        n154 = event-data() -> ()  [unwired: 1 in, 1 out]
        n155 = property on="Chart" class="WFChart (strict)"("History Data"=waveform(dbl)[][] []) -> (error out=w366:errorcluster)  [unwired: 2 in, 1 out]
        n156 = call <userlib>:"AddError.vi"("Severity"="Critical", "Priority"=u8 2, "ErrorArray In"=w368, "error in (no error)"=w366) -> ("ErrorArray Out"=w367:errorcluster[])  [unwired: 6 in, 1 out]
        n157 = property on="XY Graph" class="XYGraph (strict)"("Value"=cluster{dbl[], dbl[]} {[], []} ("XY Graph")) -> ()  [unwired: 2 in, 2 out]
      }
      event "btnReset": Value Change {
        # "Resets the Event Loops Event strucutre to handle any new events."
        n158 = event-data() -> ()  [unwired: 1 in, 1 out]
        n159 = call "ObtainBroadcastEvents.vi"() -> ("error out"=w373:errorcluster, "AcPwrEvents"=w371:T6)  [unwired: 10 in]
        n160 = register-events(reference=w382, error in=w373, w371) -> (reference out=w381:refnum<event-registration>, error out=w375:errorcluster)  [unwired: 2 in]
        n161 = property on="Chart" class="WFChart (strict)"(error in=w375, "History Data"=waveform(dbl)[][] []) -> (error out=w374:errorcluster)  [unwired: 1 in, 1 out]
        n162 = call <userlib>:"AddError.vi"("Severity"="Critical", "Priority"=u8 2, "ErrorArray In"=w380, "error in (no error)"=w374) -> ("ErrorArray Out"=w379:errorcluster[])  [unwired: 6 in, 1 out]
      }
      event "btnStop": Value Change {
        # "Stops the QMH Loop"
        n163 = event-data() -> ()  [unwired: 1 in, 1 out]
        n164 = Unbundle By Name(w385) -> ("StopRequest"=w391:refnum<user-event>)
        n165 = Generate User Event(priority (normal)=usereventprio."high priority", user event=w391, event data cluster=T14 {"BusIndex"=0, "Data"=variant} ("event data")) -> (error out=w392:errorcluster)  [unwired: 1 in, 1 out]
        n166 = call <userlib>:"AddError.vi"("Severity"="Fatal" ("String"), "Priority"=u8 0, "ErrorArray In"=w393, "error in (no error)"=w392) -> ("ErrorArray Out"=w386:errorcluster[])  [unwired: 6 in, 1 out]
      }
      event Panel Resize {
        n167 = event-data() -> ("Act"=w396:T19)  [unwired: 1 in]
        n168 = case shown="\"Minimized\"" w396 {
          tunnel: [w397 _] -> w395
          frame "Minimized" {
            n169 = local read "PluginName"() -> (w399:string)
            n170 = call "VisWindowClosed.vi"("Window Closed?"=TRUE ("Window Minimized or Clozed?"), "Module Name"=w399) -> ("error out"=w400:errorcluster)  [unwired: 9 in]
            n171 = call <userlib>:"AddError.vi"("error in (no error)"=w400) -> ("ErrorArray Out"=w397:errorcluster[])  [unwired: 9 in, 1 out]
          }
          frame "Maximized", Default {
          }
        }
      }
      event Panel Close? {
        n172 = event-data() -> ()  [unwired: 1 in, 1 out]
        n173 = local read "PluginName"() -> (w403:string)
        n174 = call "VisWindowClosed.vi"("Window Closed?"=TRUE ("Window Minimized or Clozed?"), "Module Name"=w403) -> ("error out"=w404:errorcluster)  [unwired: 9 in]
        n175 = call <userlib>:"AddError.vi"("error in (no error)"=w404) -> ("ErrorArray Out"=w402:errorcluster[])  [unwired: 9 in, 1 out]
        n176 = event-data("Discard?"=TRUE) -> ()  [unwired: 1 in, 1 out]
      }
      event Timeout {
        # "Stops the QMH Loop"
        n177 = event-data() -> ()  [unwired: 1 in, 3 out]
        n178 = call <extravilib>:"Read.vi"("channel"=w414) -> ("element"=w408:bool)  [unwired: 1 in, 1 out]
        n179 = disable-structure shown="Disabled" {
          disable-tunnel: [w419 _] -> w413
          disable-tunnel: w412 -> [w418 w431]
          disable-tunnel: w411 -> [w417 w432]
          disable-tunnel: [w416 w432] -> w410
          disable-tunnel: [w415 w431] -> w409
          frame Disabled {
            n180 = call "VisFGVStop.vi"("Error In"=w418) -> ("Error Out"=w420:errorcluster[], "Value"=w421:bool)  [unwired: 9 in]
            n181 = case shown="True" w421 {
              selector: w421 -> [w422 w425]
              tunnel: [w424 w428] -> w415
              tunnel: w420 -> [w424 w429]
              tunnel: w417 -> [w423 w427]
              tunnel: [w423 w426] -> w416
              tunnel: [w422 w425] -> w419
              frame False {
              }
              frame True {
                n182 = call "VisEnqueueElement.vi"("Priority? (F)"=w425, "Error Array In"=w429, "Message"="Stop", "queue in"=w427) -> ("Error Array Out"=w428:errorcluster[], "queue out"=w426:refnum<queue>)  [unwired: 6 in]
              }
            }
          }
          frame Enabled {
          }
        }
        n183 = Or(x=w413, y=w408) -> (x .or. y?=w407:bool)
      }
      event User Event {
        # "Checks if the measurement data received matches the PluginName control and if so sends it to the QMH loop to be displayed on the graph."
        n184 = event-data() -> ("Data"=w437:variant, "ModuleID"=w434:i32)  [unwired: 1 in]
        n185 = call <extravilib>:"Read.vi"("channel"=w436) -> ("element"=w435:bool)  [unwired: 1 in, 1 out]
        n186 = case shown="False" "btnPause" {
          tunnel: w442 -> [w450 w460]
          tunnel: w441 -> [w449 w459]
          tunnel: [w448 w459] -> w440
          tunnel: [w447 w460] -> w439
          tunnel: w437 -> [w446 _]
          tunnel: w434 -> [w443 _]
          frame False {
            n187 = Equal?(x=w443, y="ModuleID") -> (x = y?=w445:bool)
            n188 = case shown="True" w445 {
              tunnel: [w451 w457] -> w448
              tunnel: w450 -> [w452 w456]
              tunnel: w449 -> [w451 w458]
              tunnel: [w452 w454] -> w447
              tunnel: w446 -> [_ w455]
              frame False {
              }
              frame True {
                n189 = call "VisEnqueueElement.vi"("Error Array In"=w458, "Data"=w455, "Message"="Show", "queue in"=w456) -> ("Error Array Out"=w457:errorcluster[], "queue out"=w454:refnum<queue>)  [unwired: 6 in]
              }
            }
          }
          frame True {
          }
        }
      }
      event User Event {
        # "Checks if the measurement data received matches the PluginName control and if so sends it to the QMH loop to be displayed on the graph."
        n190 = event-data() -> ("Data"=w466:variant, "ModuleID"=w463:i32)  [unwired: 1 in]
        n191 = call <extravilib>:"Read.vi"("channel"=w465) -> ("element"=w464:bool)  [unwired: 1 in, 1 out]
        n192 = local read "Log Data"() -> (w462:bool)
        n193 = local read "btnPause"() -> (w461:bool)
        n194 = case shown="False" w461 {
          tunnel: w471 -> [w478 w498]
          tunnel: w470 -> [w477 w497]
          tunnel: [w476 w497] -> w469
          tunnel: [w475 w498] -> w468
          tunnel: w466 -> [w474 _]
          tunnel: w463 -> [w473 _]
          tunnel: w462 -> [w472 _]
          frame False {
            n195 = case shown="True" w472 {
              tunnel: w478 -> [w480 w488]
              tunnel: w477 -> [w479 w487]
              tunnel: [w479 w486] -> w476
              tunnel: [w480 w485] -> w475
              tunnel: w474 -> [_ w484]
              tunnel: w473 -> [_ w482]
              frame False {
              }
              frame True {
                n196 = local read "ModuleID"() -> (w481:i32)
                n197 = Equal?(x=w482, y=w481) -> (x = y?=w483:bool)
                n198 = case shown="True" w483 {
                  tunnel: [w489 w495] -> w486
                  tunnel: w488 -> [w490 w494]
                  tunnel: w487 -> [w489 w496]
                  tunnel: [w490 w492] -> w485
                  tunnel: w484 -> [_ w493]
                  frame False {
                  }
                  frame True {
                    n199 = call "VisEnqueueElement.vi"("Error Array In"=w496, "Data"=w493, "Message"="Log Parameter Set", "queue in"=w494) -> ("Error Array Out"=w495:errorcluster[], "queue out"=w492:refnum<queue>)  [unwired: 6 in]
                  }
                }
              }
            }
          }
          frame True {
          }
        }
      }
      event User Event {
        n200 = event-data() -> ("ModuleID"=w500:i32)  [unwired: 1 in, 5 out]
        n201 = local read "ModuleID"() -> (w499:i32)
        n202 = Equal?(x=w499, y=w500) -> (x = y?=w505:bool)
        n203 = case shown="True" w505 {
          tunnel: [w506 w511] -> w502
          tunnel: [w507 w510] -> w503
          tunnel: w504 -> [w507 w509]
          tunnel: w501 -> [w506 w508]
          frame False {
          }
          frame True {
            n204 = call "VisEnqueueElement.vi"("Priority? (F)"=TRUE, "Error Array In"=w508, "Message"="Stop", "queue in"=w509) -> ("Error Array Out"=w511:errorcluster[], "queue out"=w510:refnum<queue>)  [unwired: 6 in]
          }
        }
      }
      event "Display": Value Change {
        n205 = event-data() -> ("NewVal"=w517:enum16{"Raw Data", "Voltage Vs Current"})  [unwired: 1 in]
        n206 = case shown="\"Raw Data\", Default" w517 {
          tunnel: [TRUE FALSE] -> w516
          frame "Raw Data", Default {
          }
          frame "Voltage Vs Current" {
          }
        }
        n207 = Not(x=w516) -> (.not. x?=w515:bool)
        n208 = property on="Chart" class="WFChart (strict)"("Visible"=w516) -> ()  [unwired: 2 in, 2 out]
        n209 = property on="XY Graph" class="XYGraph (strict)"("Visible"=w515) -> ()  [unwired: 2 in, 2 out]
      }
      event "Voltage", "Current", "Power", "Resistance": Value Change {
        n210 = event-data() -> ("CtlRef"=w525:refnum<vi>)  [unwired: 1 in]
        n211 = property class="Bool"(reference=w525) -> ("Label.Text"=w523:string)  [unwired: 1 in, 2 out]
        n212 = call "VisEnqueueElement.vi"("Data"=w523, "Message"="Set Parameter", "queue in"=w521) -> ("Error Array Out"=w520:errorcluster[], "queue out"=w522:refnum<queue>)  [unwired: 7 in]
      }
      event "Device ON?": Value Change {
        n213 = event-data() -> ("NewVal"=w526:bool)  [unwired: 1 in]
        n214 = call "VisEnqueueElement.vi"("Data"=w526, "Message"="Device ON_OFF", "queue in"=w528) -> ("queue out"=w527:refnum<queue>)  [unwired: 7 in, 1 out]
      }
      event User Event {
        n215 = event-data() -> ("ModuleID"=w536:i32, "Data"=w530:variant)  [unwired: 1 in]
        n216 = local read "ModuleID"() -> (w537:i32)
        n217 = Equal?(x=w537, y=w536) -> (x = y?=w531:bool)
        n218 = case shown="True" w531 {
          tunnel: w535 -> [w538 w544]
          tunnel: w534 -> [w539 w543]
          tunnel: [w538 w542] -> w533
          tunnel: [w539 w541] -> w532
          tunnel: w530 -> [_ w540]
          frame False {
          }
          frame True {
            (unwired) TRUE ("Priority? (F)")
            n219 = call "VisEnqueueElement.vi"("Error Array In"=w543, "Data"=w540, "Message"="GotSettings", "queue in"=w544) -> ("Error Array Out"=w541:errorcluster[], "queue out"=w542:refnum<queue>)  [unwired: 6 in]
          }
        }
      }
      event "btnStopModule": Value Change {
        n220 = event-data() -> ()  [unwired: 1 in, 1 out]
        n221 = local read "ModuleID"() -> (w548:i32)
        n222 = call "StatusUpdateByModID.vi"("Status"="User requested module stop", "Accessors:Module ID"=w548) -> ("error out"=w549:errorcluster)  [unwired: 9 in]
        n223 = flat-sequence {
          tunnel: [w552] -> w550
          tunnel: w549 -> [_]
          frame #0 {
            n224 = local read "PluginName"() -> (w551:string)
            n225 = call "GetSetTestClass.vi"() -> ("Test.lvclass"=w553:refnum<class "Test.lvclass">)  [unwired: 11 in]
            n226 = call "StopModByName.vi"("Module Name"=w551, "Test.lvclass"=w553) -> ("ErrorArray Out"=w552:errorcluster[])  [unwired: 4 in, 5 out]
          }
        }
      }
      event User Event {
        # "Framework requested visualization stop"
        n227 = event-data() -> ("Data"=w554:variant)  [unwired: 1 in]
        n228 = local read "PluginName"() -> (w555:string)
        n229 = Variant To Data(type="" ("Message"), Variant=w554) -> (data=w565:string, error out=w563:errorcluster)  [unwired: 1 in]
        n230 = call <userlib>:"AddError.vi"("Severity"="Inform", "Priority"=u8 3, "ErrorArray In"=w558, "error in (no error)"=w563) -> ("ErrorArray Out"=w562:errorcluster[])  [unwired: 6 in, 1 out]
        n231 = Equal?(x=w555, y=w565) -> (x = y?=w564:bool)
        n232 = case shown="False" w564 {
          tunnel: w559 -> [w568 w572]
          tunnel: [w567 w571] -> w557
          tunnel: w562 -> [w567 w570]
          tunnel: [w568 w569] -> w556
          frame False {
          }
          frame True {
            n233 = call "VisEnqueueElement.vi"("Priority? (F)"=TRUE, "Error Array In"=w570, "Message"="Stop", "queue in"=w572) -> ("Error Array Out"=w571:errorcluster[], "queue out"=w569:refnum<queue>)  [unwired: 6 in]
          }
        }
      }
      event "Chart": Shortcut Menu Activation? {
        n234 = event-data() -> ("CtlRef"=w581:refnum<vi>, "MenuRef"=w580:refnum<k9>, "Coords"=w579:T20)  [unwired: 1 in]
        n235 = local read "MeasChannels"() -> (w578:string[])
        n236 = call "Handle Chart Menu Activation.vi"("Channel Names"=w578, "Coords"=w579, "MenuRef"=w580, "CtlRef"=w581) -> ("Channel Index"=→"Chart#":i32)  [unwired: 7 in]
        n237 = event-data() -> ()  [unwired: 2 in, 1 out]
      }
      event "Chart": Shortcut Menu Selection (User) {
        n238 = event-data() -> ("ItemTag"=w582:string)  [unwired: 1 in, 1 out]
        n239 = Match Pattern(string=w582, regular expression="Meas_") -> (after substring=w588:string, offset past match=w589:i32)  [unwired: 1 in, 2 out]
        n240 = case shown="Default" w589 {
          tunnel: w584 -> [w594 w597]
          tunnel: w583 -> [w593 w596]
          tunnel: [w592 w597] -> w586
          tunnel: [w591 w596] -> w585
          tunnel: w588 -> [w590 _]
          frame Default {
            # "User selected a measurement variable\nin the Chart shortcut menu"
            n241 = call "VisEnqueueElement.vi"("Error Array In"=w593, "Data"=w590, "Message"="Meas Variable Changed", "queue in"=w594) -> ("Error Array Out"=w591:errorcluster[], "queue out"=w592:refnum<queue>)  [unwired: 6 in]
          }
          frame -1 {
          }
        }
      }
    }
    n242 = call "VisEnqueueError.vi"("Error Array In"=w354, "Queue in"=w353) -> ("Error Array Out"=w355:errorcluster[], "Queue out"=w352:refnum<queue>)  [unwired: 8 in]
  }
  n243 = while {
    stop <- w598 stop-if-true
    # "Loop Parameters"
    n244 = event shown="[0] \"btnRunParamLoop\": Value Change" {
      selector: _ -> [_ _ _ _ _]
      dyn-events: _ -> [_ _ _ _ _]
      timeout: _ -> [_ _ _ _ _]
      tunnel: [_ _ _ _ TRUE] -> w598
      event "btnRunParamLoop": Value Change {
        # "AcPwrLoopParameter,DC,Voltage,-1,7.5,0.25,2,5,#"
        # "Send parameter looping script"
        n245 = event-data() -> ()  [unwired: 1 in, 1 out]
        n246 = local read "CurrentType"() -> (w611:string)
        n247 = local read "Loop Parameters"() -> (w612:T1)
        n248 = local read "PluginName"() -> (w604:string)
        n249 = Unbundle By Name(w612) -> ("Parameter"=w610:T21, "Start Value"=w609:dbl, "Increment"=w608:dbl, "Interval (s)"=w607:dbl, "# Iterations"=w606:u32)
        n250 = Match Pattern(string=w604, regular expression="[.]") -> (after substring=w600:string)  [unwired: 1 in, 3 out]
        n251 = Format Into String(format string="AcPwrLoopParameter,%s,%s,-1,%#4g,%#4f,%#4g,%d,#%s", w611, w610, w609, w608, w607, w606, w600) -> (resulting string=w599:string)  [unwired: 2 in, 1 out]
        n252 = invoke class="App" method="Clipboard.Write"("Param 0"=w599) -> ()  [unwired: 3 in, 4 out]
        n253 = call "GetSetTestClass.vi"() -> ("Test.lvclass"=w601:refnum<class "Test.lvclass">)  [unwired: 11 in]
        n254 = Build Array(w599, "Stop" ("element")) -> (w602:string[])
        n255 = call "ScriptedStateMachine.vi"("script"=w602, "Test.lvclass 2"=w601) -> ()  [unwired: 7 in, 3 out]
      }
      event "btnStopParameterLoop": Value Change {
        n256 = event-data() -> ()  [unwired: 1 in, 6 out]
      }
      event Value Change {
        n257 = event-data() -> ()  [unwired: 1 in, 1 out]
        n258 = Unbundle By Name("Loop Parameters") -> ("End Value"=w621:dbl, "Start Value"=w620:dbl, "# Iterations"=w618:u32)
        n259 = Decrement(x=w618) -> (x-1=w615:u32)
        n260 = Subtract(x=w621, y=w620) -> (x-y=w619:dbl)
        n261 = Divide(x=w619, y=w615) -> (x/y=w617:dbl)
        n262 = Bundle By Name(cluster="Loop Parameters", "Increment"=w617) -> (w616:T1)
        n263 = local write "Loop Parameters"(w616) -> ()
      }
      event Value Change {
        n264 = event-data() -> ()  [unwired: 1 in, 1 out]
        n265 = local read "Loop Parameters"() -> (w627:T1)
        n266 = Unbundle By Name(w627) -> ("End Value"=w630:dbl, "Start Value"=w629:dbl, "Increment"=w624:dbl)
        n267 = Subtract(x=w630, y=w629) -> (x-y=w628:dbl)
        n268 = Divide(x=w628, y=w624) -> (x/y=w626:dbl)
        n269 = Round Toward -Infinity(1:w626) -> (0:w623:dbl)
        n270 = Increment(x=w623) -> (x+1=w622:dbl)
        n271 = Bundle By Name(cluster=w627, "# Iterations"=w622) -> (w625:T1)
        n272 = local write "Loop Parameters"(w625) -> ()
      }
      event "ExitHelperLoops?": Value Change {
        n273 = event-data() -> ()  [unwired: 1 in, 1 out]
      }
    }
  }
  n274 = Unregister For Events(event registration refnum=w40) -> (error out=w38:errorcluster)  [unwired: 1 in]
  n275 = flat-sequence {
    tunnel: w38 -> [w635]
    tunnel: [w634] -> w36
    tunnel: w23 -> [w633]
    tunnel: w13 -> [_]
    frame #0 {
      n276 = Release Queue(queue=w633, force destroy? (F)=TRUE, error in (no error)=w635) -> (error out=w634:errorcluster)  [unwired: 2 out]
    }
  }
  n277 = Build Array (concatenate)(w39, w13) -> (w37:errorcluster[])
  n278 = flat-sequence {
    tunnel: w13 -> [_]
    tunnel: w2 -> [w636]
    frame #0 {
      n279 = TDMS Close(11:w636) -> ()  [unwired: 1 in, 2 out]
      n280 = property on="ExitHelperLoops?" class="Bool (strict)"("Val(Sgnl)"=TRUE ("Value (Signaling)")) -> ()  [unwired: 2 in, 2 out]
    }
  }
  n281 = call <userlib>:"AddError.vi"("ErrorArray In"=w37, "error in (no error)"=w36) -> ("ErrorArray Out"=w35:errorcluster[])  [unwired: 8 in, 1 out]
  n282 = disable-structure shown="Disabled" {
    disable-tunnel: w35 -> [w640 w646]
    disable-tunnel: w34 -> [w639 _]
    disable-tunnel: [w638 w646] -> w10
    frame Disabled {
      n283 = Cluster To Array(cluster=w639) -> (array=w641:refnum<user-event>[])
      n284 = for {
        tunnel: w641 -> [w645] mode=indexing
        shift-right: [w644] -> w638
        shift-left: w640 -> [w643]
        n285 = Destroy User Event(user event=w645) -> (error out=w642:errorcluster)  [unwired: 1 in]
        n286 = call <userlib>:"AddError.vi"("ErrorArray In"=w643, "error in (no error)"=w642) -> ("ErrorArray Out"=w644:errorcluster[])  [unwired: 8 in, 1 out]
      }
    }
    frame Enabled {
    }
  }
  "ErrorArray" <- w10
  n287 = Empty Array?(array=w10) -> (empty?=w33:bool)
  n288 = flat-sequence {
    tunnel: "PluginName" -> [w648]
    tunnel: w10 -> [_]
    frame #0 {
      n289 = call "VisDidStop.vi"("DidStop?"=TRUE, "Module Name"=w648) -> ()  [unwired: 9 in, 1 out]
    }
  }
  n290 = case shown="True" w33 {
    tunnel: [w649 _] -> w22
    tunnel: w10 -> [w650 _]
    frame False {
      n291 = Merge Errors(w650) -> (w649:errorcluster)
    }
    frame True {
      n292 = invoke class="VI" method="FP.Close"() -> ()  [unwired: 3 in, 3 out]
    }
  }
  n293 = call <vilib>:"Simple Error Handler.vi"("error in (no error)"=w22) -> ()  [unwired: 4 in, 5 out]
